vi "VeriStand DSF.Transfer.Configuration.Verify.Contiguous Engine Offsets.vi"(8 "error in (no error)":errorcluster, 11 "channel configurations":T1[](array[typedef]) {"count" format="%d bytes"}) -> (0 "error out":errorcluster)   [LabVIEW 2017, in "Data Sharing Custom Device Engine.lvlib" / "VeriStand DSF.Transfer.Configuration.lvclass"]
uses:
  VeriStand DSF.Transfer.Configuration.lvclass
  Builds/Data Sharing Framework/Current/Data Sharing Framework Core/DSF Core.lvlibp/DSF Configuration API/Public/Controls/DSF Engine Channel Configuration.ctl
  Builds/Data Sharing Framework/Current/Data Sharing Framework Core/DSF Core.lvlibp/DSF Configuration API/Public/Controls/DSF Data Type.ctl
  Builds/Data Sharing Framework/Current/Data Sharing Framework Core/DSF Core.lvlibp/DSF Configuration API/Public/Controls/DSF Settings Info.ctl
  Builds/Data Sharing Framework/Current/Data Sharing Framework Core/DSF Core.lvlibp
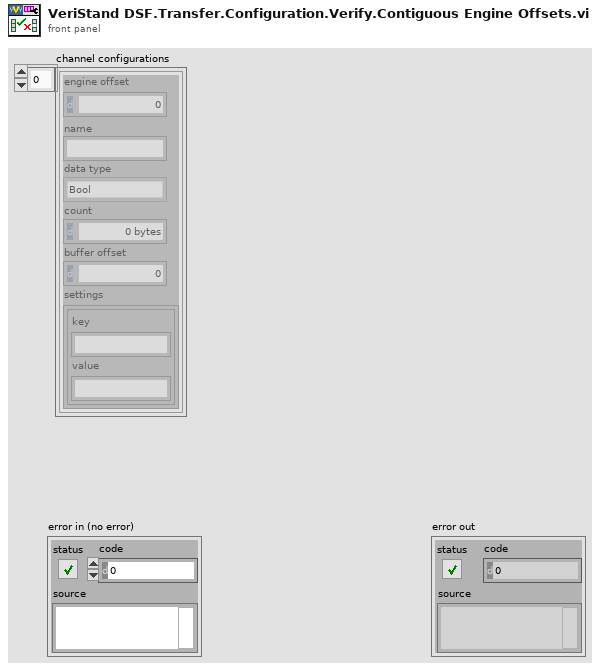
[diagram p1: front panel]
types:
  T1 = typedef "DSF Core.lvlibp/DSF Engine Channel Configuration.ctl" = cluster{"engine offset":u64, "name":string, "data type":T2, "count":u64, "buffer offset":u64, "settings":T3}
  T2 = typedef "DSF Core.lvlibp/DSF Data Type.ctl" = enum8{"Bool", "SGL", "DBL", "I8", "I16", "I32", "I64", "U8", "U16", "U32", "U64"}
  T3 = typedef "DSF Core.lvlibp/DSF Settings Info.ctl" = cluster{"key":string, "value":string}[]
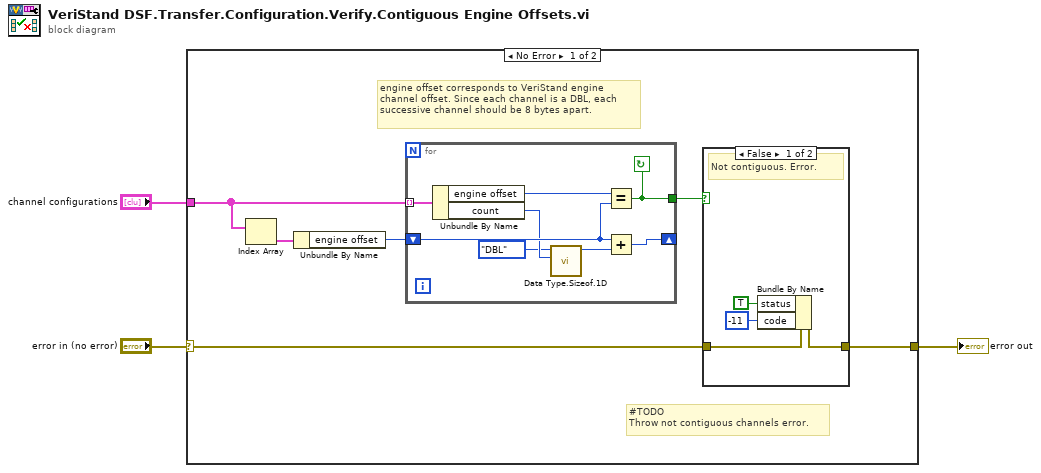
[diagram p0: block diagram]
diagram:
  n1 = case shown="No Error" "error in (no error)" {
    selector: "error in (no error)" -> [w4 w23]
    tunnel: "channel configurations" -> [w9 _]
    tunnel: [w5 w23] -> w2
    frame No Error {
      # "#TODO\nThrow not contiguous channels error."
      # "engine offset corresponds to VeriStand engine channel offset. Since each channel is a DBL, each successive channel should be 8 bytes apart."
      n2 = Index Array(array=w9) -> (element=w7:T1)  [unwired: 1 in]
      n3 = Unbundle By Name(w7) -> ("engine offset"=w8:u64)
      n4 = for {
        shift-right: [w18] -> _
        shift-left: w8 -> [w20]
        tunnel: w9 -> [w22] mode=indexing
        tunnel: [w19] -> w6
        stop <- w19 continue-if-true
        n5 = Unbundle By Name(w22) -> ("engine offset"=w21:u64, "count"=w16:u64)
        n6 = call "Data Type.Sizeof.1D.vi"("count"=w16, "data type"=DSF_Data_Type."DBL") -> ("size in bytes"=w17:u64)  [unwired: 9 in]
        n7 = Equal?(x=w21, y=w20) -> (x = y?=w19:bool)
        n8 = Add(x=w20, y=w17) -> (x+y=w18:u64)
      }
      n9 = case shown="False" w6 {
        tunnel: w4 -> [w13 w14]
        tunnel: [w10 w14] -> w5
        frame False {
          # "Not contiguous. Error."
          n10 = Bundle By Name(cluster=w13, "status"=TRUE, "code"=-11) -> (w10:errorcluster)
        }
        frame True {
          # "Contiguous. Proceed."
        }
      }
    }
    frame Error {
    }
  }
  "error out" <- w2
